vi "PC-Main.vi"() -> ()   [LabVIEW 2017]
doc: "The PC-Based PC-Main programme is a TCP/IP capable controller design to connect to the MR-Main programme in order to pass and receive data to simulate customisable cooling and emergency events via control of the MyRIO attached hardware, such as a PWM servo.\nIt has limited functionality if not connected to thge MR-Main programme."
uses:
  <vilib>/vision/Image Controls.llb/IMAQ Image.ctl
panel:
  out "Temperature (C)":dbl(knob) scale=18.0..30.0 scale format="%#.2g"
  out "Console":string
  out "Cool System Off Log":bool
  out "Z-Value\n(Debug)":dbl
  out "Y-Value\n(Debug":dbl
  out "X-Value\n(Debug)":dbl
  out "High Temp Log":bool
  out "Cool System On Log":bool
  out "Cool 4 Log":bool
  out "Cool 3 Log":bool
  out "Cool 2 Log":bool
  out "Cool 1 Log":bool
  out "Destroyed Log":bool
  out "Local Log":bool
  out "Moved Log":bool
  out "Disconnect Log":bool
  out "Connection Log":bool
  out "Nom Temp Log":bool
  out "Event Status\n(Debug)":u8
  out "User Level\n(Debug)":i32
  out "Local Request":bool
  out "Self Destruct":bool
  out "Master Warning":bool
  out "Cooling System":string
  in  "Auth":bool
  in  "Auth 2":bool
  in  "Authorise\nMovement (Debug)":bool
  out "Image":T1(plugin-control)
  out "Connected":bool
  out "Watchdog\n(Debug)":u8
  out "Net Error Source\n(Debug)":string
  out "Net Error Code\n(Debug)":i32
  out "Net Error Status\n(Debug)":bool
  in  "Quit":bool
  out "Handler Error Code\n(Debug)":i32
  in  "Cooling\nSwitch":bool
  out "Status System":timestamp format="%<%H:%M:%S\n%Y/%m/%d>T"
  out "Cooling Event Array\n(Debug)":bool[](array[boolean])
  out "Data Size\n(Debug)":i32
  out "String Length\n(Debug)":i32
  out "Cooling System Status":bool
  out "Cool Ind 4":bool
  out "Cool Ind 3":bool
  out "Cool Ind 2":bool
  out "Cool Ind 1":bool
  in  "Log Off":bool
  out "Movement":cluster{dbl, dbl, dbl}(graph)
  out "User Status":string
  in  "Password Match\n(Debug)":string[](array[string])
  in  "User Type\n(Debug)":string[](array[string])
  in  "Login":bool
  in  "Cooling 4 Off":timestamp format="%<%H:%M:%S>T"
  in  "Cooling 4 On":timestamp format="%<%H:%M:%S>T"
  in  "Cooling 3 Off":timestamp format="%<%H:%M:%S>T"
  in  "Cooling 3 On":timestamp format="%<%H:%M:%S>T"
  in  "Cooling 2 Off":timestamp format="%<%H:%M:%S>T"
  in  "Cooling 2 On":timestamp format="%<%H:%M:%S>T"
  in  "Cooling 1 Off":timestamp format="%<%H:%M:%S>T"
  in  "Cooling 1 On":timestamp format="%<%H:%M:%S>T"
  in  "Password":string
  in  "Username":string
  out "System Status":string
  out "Emergency Cooling":bool
  out "Safe System Temperature":bool
  # "Sensor System"
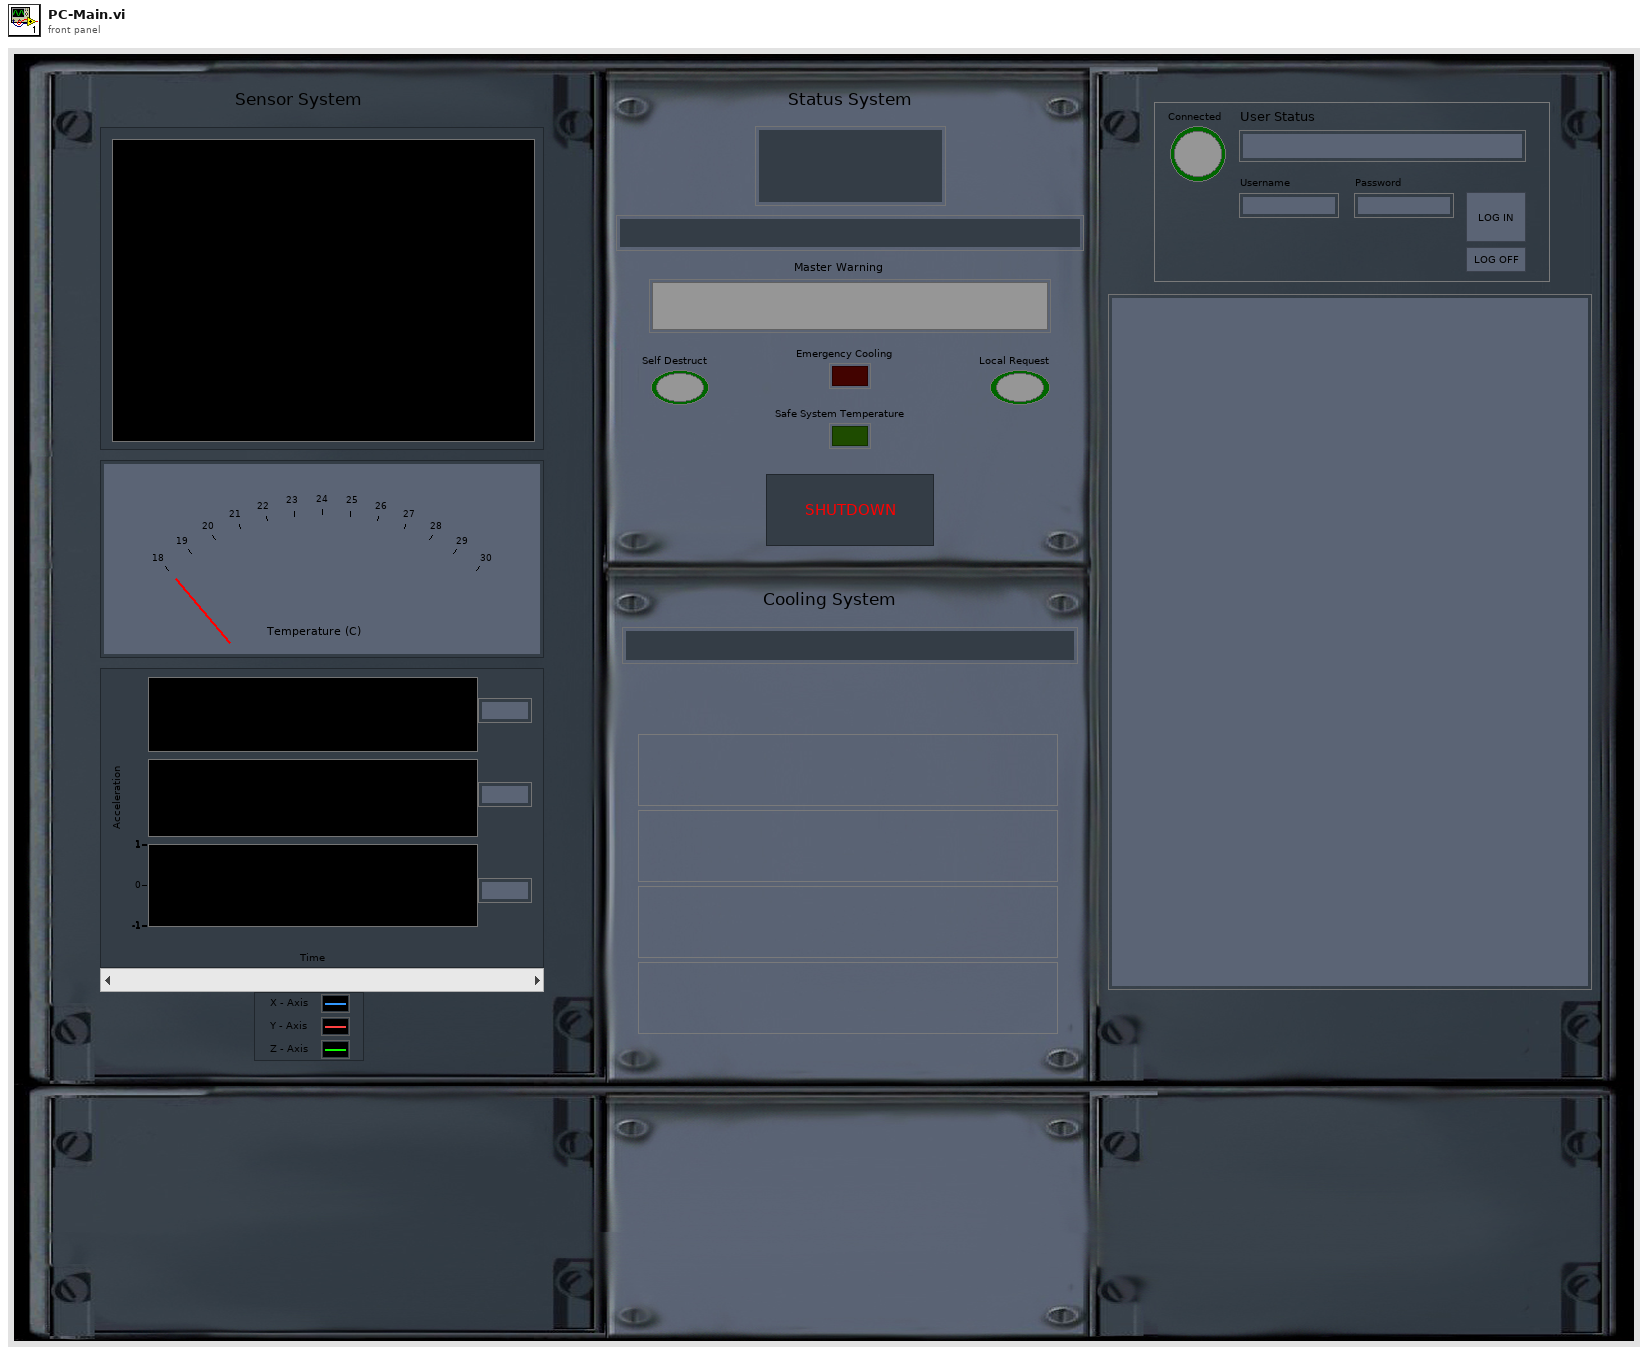
[diagram p1: front panel]
types:
  T1 = typedef "IMAQ Image.ctl" = refnum<image>
  T2 = cluster{"Numeric":dbl, "Knob":dbl, "Knob 2":dbl, "Knob 3":dbl, bool, "bytes to read":u8, "bytes to read 2":u8}
  T3 = cluster{"Numeric":dbl, "Numeric":dbl, "Numeric":dbl}
  T4 = cluster{"Cool Ind 1":bool, "Cool Ind 2":bool, "Cool Ind 3":bool, "Cool Ind 4":bool, bool, dbl, "Authorise\nMovement (Debug)":bool}
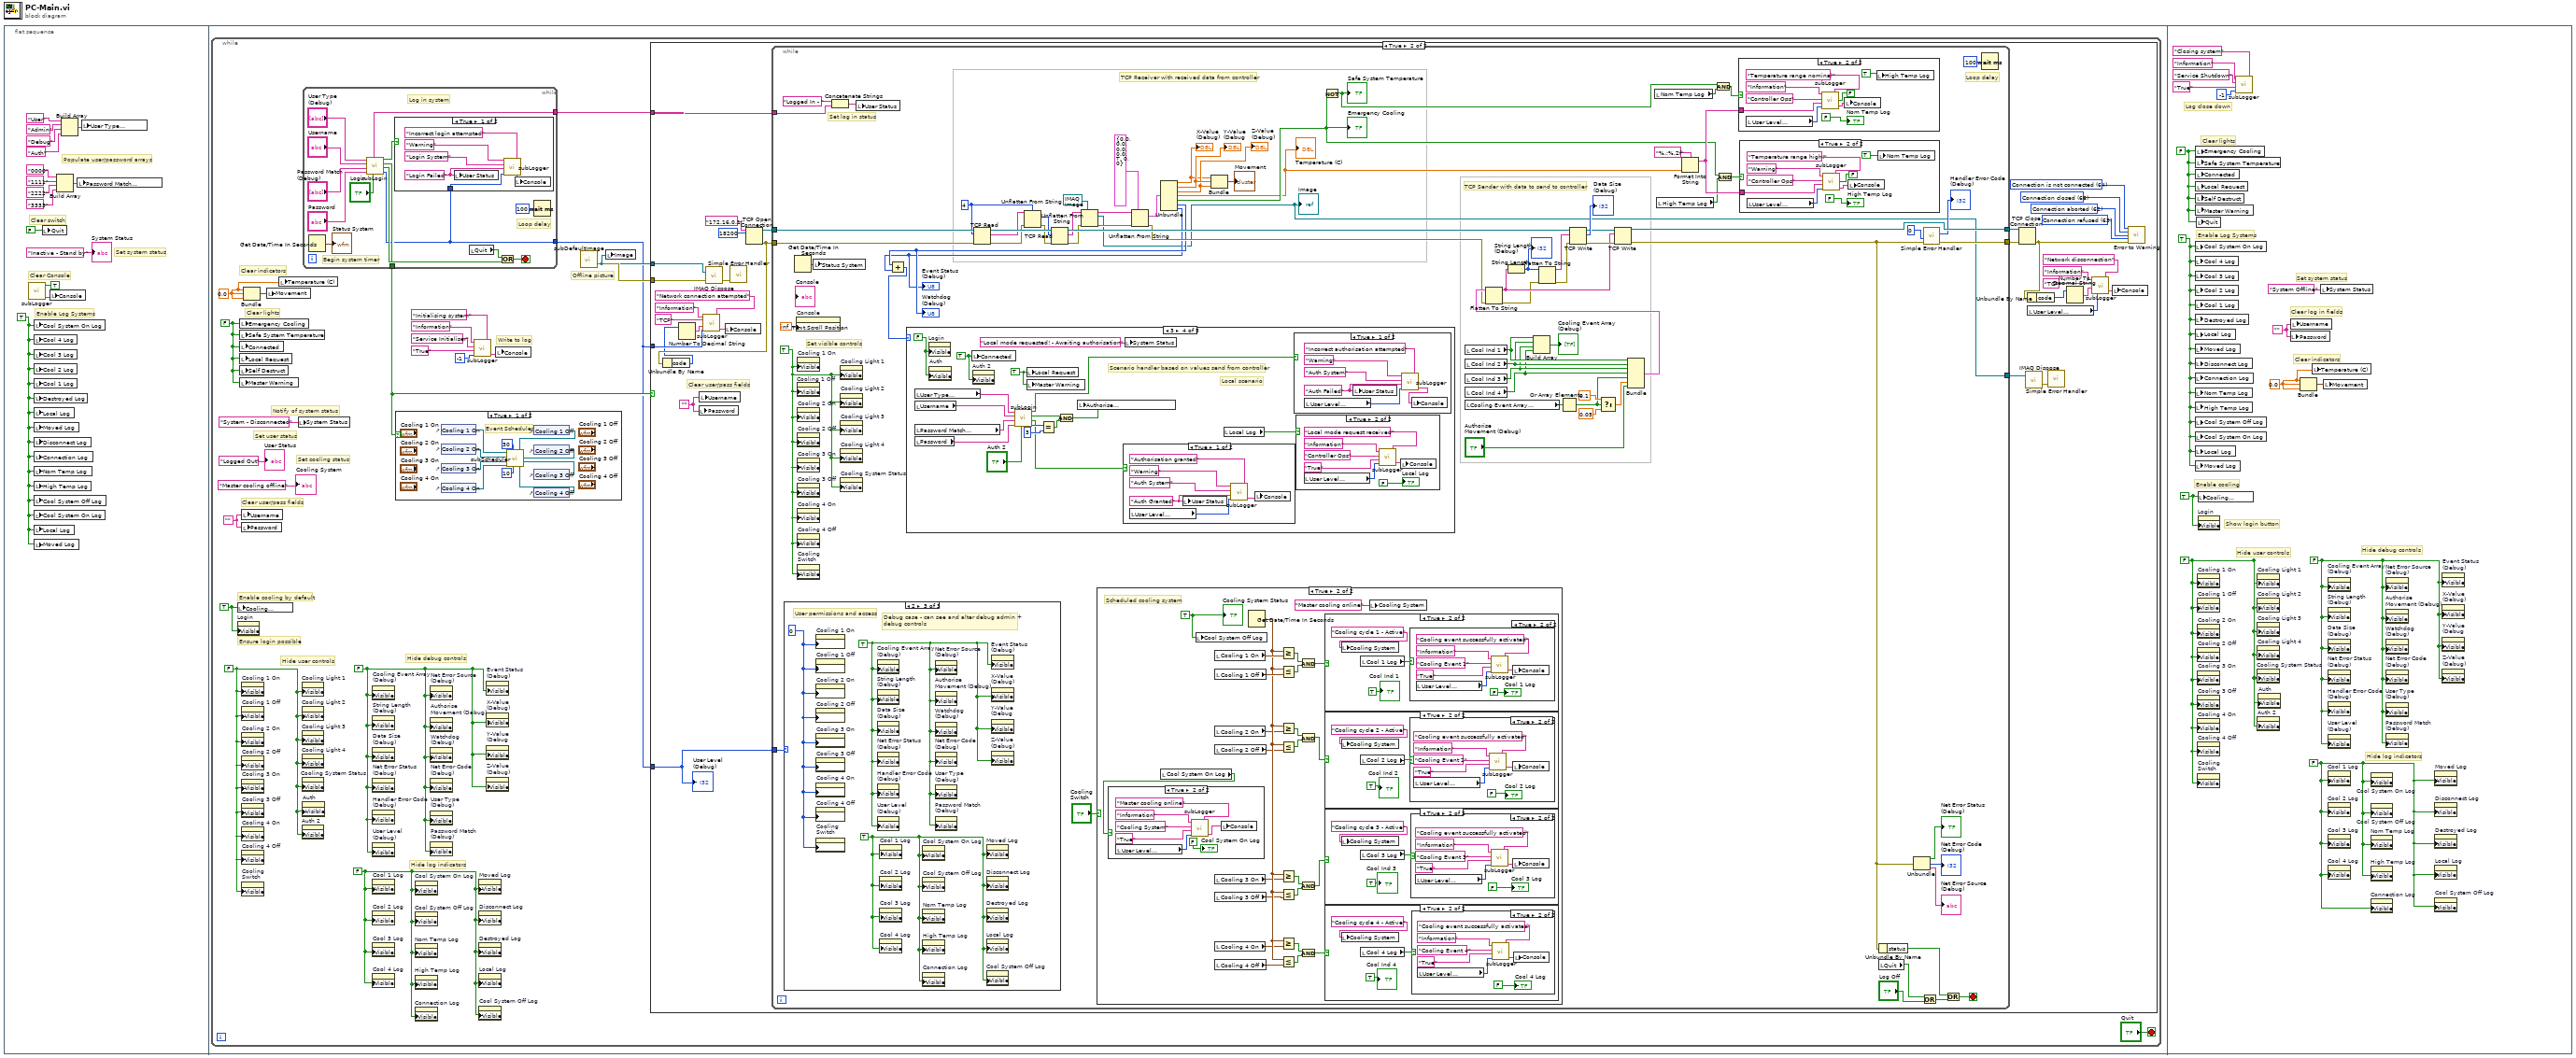
[diagram p0: block diagram]
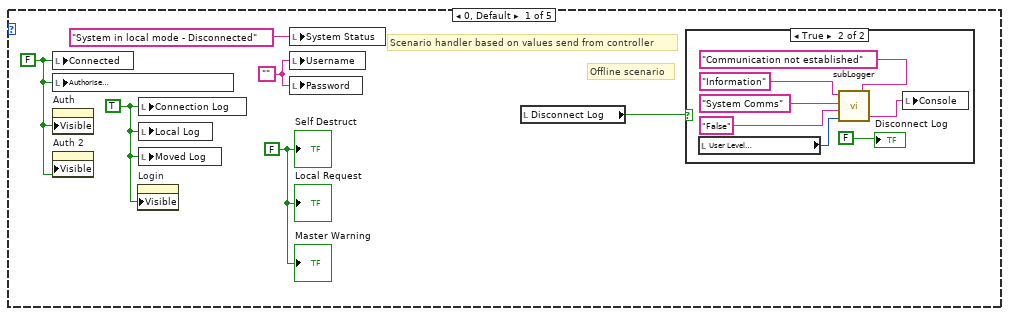
[diagram p7: hidden frame]
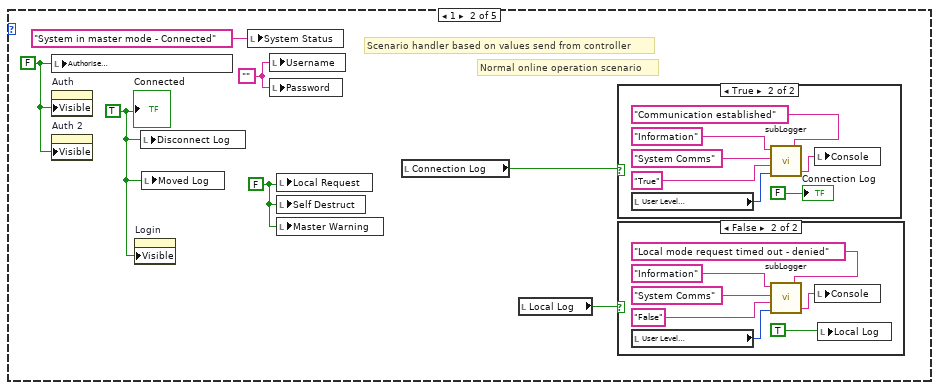
[diagram p9: hidden frame]
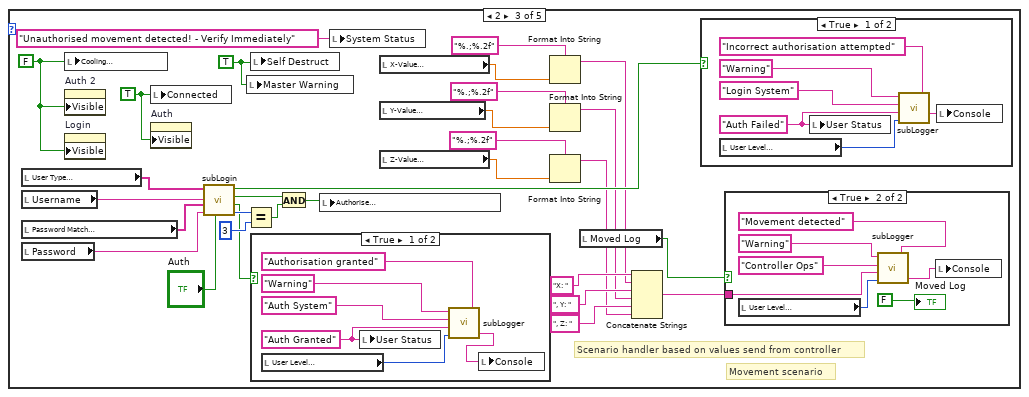
[diagram p12: hidden frame]
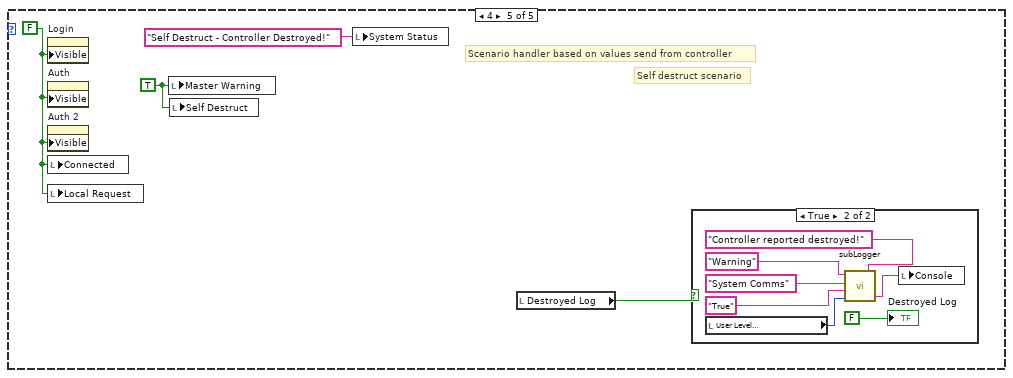
[diagram p19: hidden frame]
diagram:
  n1 = flat-sequence {
    frame #0 {
      w3 = TRUE
      # "Clear Console"
      # "Enable Log Systems"
      # "Set system status"
      # "Clear switch"
      # "Populate user/password arrays"
      n2 = call "subLogger.vi"("Clear Flag"=TRUE) -> ("To Screen"=w2:string)  [unwired: 5 in]
      n3 = local write "Cool System On Log"(w3) -> ()
      n4 = local write "Cool 4 Log"(w3) -> ()
      n5 = local write "Cool 3 Log"(w3) -> ()
      n6 = local write "Cool 2 Log"(w3) -> ()
      n7 = local write "Cool 1 Log"(w3) -> ()
      n8 = local write "Destroyed Log"(w3) -> ()
      n9 = local write "Local Log"(w3) -> ()
      n10 = local write "Moved Log"(w3) -> ()
      n11 = local write "Disconnect Log"(w3) -> ()
      n12 = local write "Connection Log"(w3) -> ()
      n13 = local write "Nom Temp Log"(w3) -> ()
      n14 = local write "High Temp Log"(w3) -> ()
      n15 = local write "Cool System Off Log"(w3) -> ()
      n16 = local write "Cool System On Log"(w3) -> ()
      n17 = local write "Local Log"(w3) -> ()
      n18 = local write "Moved Log"(w3) -> ()
      n19 = local write "Quit"(FALSE) -> ()
      n20 = local write "Console"(w2) -> ()
      n21 = Build Array("0000", "1111", "2222", "3333") -> (w15:string[])
      n22 = Build Array("User", "Admin", "Debug", "Auth") -> (w14:string[])
      n23 = local write "Password Match\n(Debug)"(w15) -> ()
      n24 = local write "User Type\n(Debug)"(w14) -> ()
      "System Status" <- "Inactive - Stand by"
    }
    frame #1 {
      n25 = while {
        stop <- "Quit" stop-if-true
        w17 = FALSE
        w18 = FALSE
        w33 = ""
        w16 = 0.0 ("Numeric")
        w27 = FALSE
        w31 = TRUE
        w19 = FALSE
        # "Offline picture"
        # "Hide log indicators"
        # "Hide debug controls"
        # "Write to log"
        # "Set cooling status"
        # "Ensure login possible"
        # "Notify of system status"
        # "Clear user/pass fields"
        # "Clear lights"
        # "Clear indicators"
        # "Enable cooling by default"
        # "Set user status"
        # "Hide user controls"
        n26 = local write "Cooling\nSwitch"(w31) -> ()
        n27 = property on="Login" class="Bool"("Visible"=w31) -> ()  [unwired: 2 in, 2 out]
        n28 = local write "Emergency Cooling"(w27) -> ()
        n29 = local write "Safe System Temperature"(w27) -> ()
        n30 = local write "Connected"(w27) -> ()
        n31 = local write "Local Request"(w27) -> ()
        n32 = local write "Self Destruct"(w27) -> ()
        n33 = local write "Master Warning"(w27) -> ()
        n34 = local write "Username"(w33) -> ()
        n35 = local write "Password"(w33) -> ()
        n36 = property on="Cooling 1 On" class="AbsTime (strict)"("Visible"=w19) -> ()  [unwired: 2 in, 2 out]
        n37 = property on="Cooling 1 Off" class="AbsTime (strict)"("Visible"=w19) -> ()  [unwired: 2 in, 2 out]
        n38 = property on="Cooling 2 On" class="AbsTime (strict)"("Visible"=w19) -> ()  [unwired: 2 in, 2 out]
        n39 = property on="Cooling 2 Off" class="AbsTime (strict)"("Visible"=w19) -> ()  [unwired: 2 in, 2 out]
        n40 = property on="Cooling 3 On" class="AbsTime (strict)"("Visible"=w19) -> ()  [unwired: 2 in, 2 out]
        n41 = property on="Cooling 3 Off" class="AbsTime (strict)"("Visible"=w19) -> ()  [unwired: 2 in, 2 out]
        n42 = property on="Cooling 4 On" class="AbsTime (strict)"("Visible"=w19) -> ()  [unwired: 2 in, 2 out]
        n43 = property on="Cooling 4 Off" class="AbsTime (strict)"("Visible"=w19) -> ()  [unwired: 2 in, 2 out]
        n44 = property on="Cooling\nSwitch" class="Bool (strict)"("Visible"=w19) -> ()  [unwired: 2 in, 2 out]
        n45 = Bundle("Numeric"=w16, "Numeric"=w16, "Numeric"=w16) -> (w34:T3)  [unwired: 1 in]
        n46 = local write "Movement"(w34) -> ()
        n47 = local write "Temperature (C)"(w16) -> ()
        n48 = local write "System Status"("System - Disconnected") -> ()
        n49 = property on="Cooling Light 1" class="Bool (strict)"("Visible"=w19) -> ()  [unwired: 2 in, 2 out]
        n50 = property on="Cooling Light 2" class="Bool (strict)"("Visible"=w19) -> ()  [unwired: 2 in, 2 out]
        n51 = property on="Cooling Light 3" class="Bool (strict)"("Visible"=w19) -> ()  [unwired: 2 in, 2 out]
        n52 = property on="Cooling Light 4" class="Bool (strict)"("Visible"=w19) -> ()  [unwired: 2 in, 2 out]
        n53 = property on="Cooling System Status" class="Bool (strict)"("Visible"=w19) -> ()  [unwired: 2 in, 2 out]
        n54 = property on="Auth 2" class="Bool"("Visible"=w19) -> ()  [unwired: 2 in, 2 out]
        n55 = property on="Auth" class="Bool"("Visible"=w19) -> ()  [unwired: 2 in, 2 out]
        n56 = while {
          tunnel: [w50] -> w26
          tunnel: [w56] -> w37
          tunnel: [w59] -> w38
          stop <- w62 stop-if-true
          # "Log in system"
          # "Loop delay"
          # "Begin system timer"
          n57 = Get Date/Time In Seconds() -> (seconds since 1Jan1904=→"Status System":timestamp)
          n58 = call "subLogin.vi"("Login Button"="Login", "Password Entry"="Password", "Password Array"="Password Match\n(Debug)", "User Entry"="Username", "User Array"="User Type\n(Debug)") -> ("Array Index No"=w50:i32, "If Correct 2"=w57:bool, "If Correct 1"=w56:bool, "If Incorrect"=w58:bool, "Username Out"=w59:string)
          n59 = case shown="True" w58 {
            tunnel: w50 -> [w65 _]
            frame True {
              w66 = "Login Failed"
              n60 = local write "User Status"(w66) -> ()
              n61 = call "subLogger.vi"("Description"="Incorrect login attempted", "User Level"=w65, "Value"=w66, "Location"="Login System", "Level"="Warning") -> ("To Screen"=w63:string)  [unwired: 1 in]
              n62 = local write "Console"(w63) -> ()
            }
            frame False {
            }
          }
          n63 = local read "Quit"() -> (w61:bool)
          n64 = Or(x=w61, y=w57) -> (x .or. y?=w62:bool)
          n65 = Wait (ms)(milliseconds to wait=u32 100) -> ()  [unwired: 1 out]
        }
        n66 = property on="Cooling Event Array\n(Debug)" class="Arr (strict)"("Visible"=w17) -> ()  [unwired: 2 in, 2 out]
        n67 = property on="String Length\n(Debug)" class="DigNum (strict)"("Visible"=w17) -> ()  [unwired: 2 in, 2 out]
        n68 = property on="Data Size\n(Debug)" class="DigNum (strict)"("Visible"=w17) -> ()  [unwired: 2 in, 2 out]
        n69 = property on="Net Error Status\n(Debug)" class="Bool (strict)"("Visible"=w17) -> ()  [unwired: 2 in, 2 out]
        n70 = property on="Handler Error Code\n(Debug)" class="DigNum (strict)"("Visible"=w17) -> ()  [unwired: 2 in, 2 out]
        n71 = property on="User Level\n(Debug)" class="DigNum (strict)"("Visible"=w17) -> ()  [unwired: 2 in, 2 out]
        n72 = property on="Cool 1 Log" class="Bool (strict)"("Visible"=w18) -> ()  [unwired: 2 in, 2 out]
        n73 = property on="Cool 2 Log" class="Bool (strict)"("Visible"=w18) -> ()  [unwired: 2 in, 2 out]
        n74 = property on="Cool 3 Log" class="Bool (strict)"("Visible"=w18) -> ()  [unwired: 2 in, 2 out]
        n75 = property on="Cool 4 Log" class="Bool (strict)"("Visible"=w18) -> ()  [unwired: 2 in, 2 out]
        n76 = case shown="True" w37 {
          frame True {
            # "Event Scheduler"
            n77 = control-ref of="Cooling 1 On"() -> (w42:refnum<vi>)
            n78 = control-ref of="Cooling 2 On"() -> (w41:refnum<vi>)
            n79 = control-ref of="Cooling 3 On"() -> (w40:refnum<vi>)
            n80 = control-ref of="Cooling 4 On"() -> (w39:refnum<vi>)
            n81 = control-ref of="Cooling 1 Off"() -> (w46:refnum<vi>)
            n82 = control-ref of="Cooling 2 Off"() -> (w45:refnum<vi>)
            n83 = control-ref of="Cooling 3 Off"() -> (w44:refnum<vi>)
            n84 = control-ref of="Cooling 4 Off"() -> (w43:refnum<vi>)
            n85 = call "subScheduler.vi"("Cooling 4 Off"=w43, "Cooling 3 Off"=w44, "Cooling 2 Off"=w45, "Cooling 1 Off"=w46, "Deactivate Offset"=10, "Activate Offset"=30, "Cooling 4 On"=w39, "Cooling 3 On"=w40, "Cooling 2 On"=w41, "Cooling 1 On"=w42) -> ()
          }
          frame False {
            # "Event Scheduler"
          }
        }
        n86 = property on="Cool System On Log" class="Bool (strict)"("Visible"=w18) -> ()  [unwired: 2 in, 2 out]
        n87 = property on="Cool System Off Log" class="Bool (strict)"("Visible"=w18) -> ()  [unwired: 2 in, 2 out]
        n88 = property on="Nom Temp Log" class="Bool (strict)"("Visible"=w18) -> ()  [unwired: 2 in, 2 out]
        n89 = property on="High Temp Log" class="Bool (strict)"("Visible"=w18) -> ()  [unwired: 2 in, 2 out]
        n90 = property on="Connection Log" class="Bool (strict)"("Visible"=w18) -> ()  [unwired: 2 in, 2 out]
        n91 = property on="Net Error Source\n(Debug)" class="Str"("Visible"=w17) -> ()  [unwired: 2 in, 2 out]
        n92 = property on="Authorise\nMovement (Debug)" class="Bool (strict)"("Visible"=w17) -> ()  [unwired: 2 in, 2 out]
        n93 = property on="Watchdog\n(Debug)" class="DigNum (strict)"("Visible"=w17) -> ()  [unwired: 2 in, 2 out]
        n94 = property on="Net Error Code\n(Debug)" class="DigNum (strict)"("Visible"=w17) -> ()  [unwired: 2 in, 2 out]
        n95 = property on="User Type\n(Debug)" class="Arr (strict)"("Visible"=w17) -> ()  [unwired: 2 in, 2 out]
        n96 = property on="Password Match\n(Debug)" class="Arr (strict)"("Visible"=w17) -> ()  [unwired: 2 in, 2 out]
        n97 = call "subLogger.vi"("Description"="Initialising system", "User Level"=-1, "Value"="True", "Location"="Service Initialiser", "Level"="Information") -> ("To Screen"=w25:string)  [unwired: 1 in]
        n98 = property on="Moved Log" class="Bool (strict)"("Visible"=w18) -> ()  [unwired: 2 in, 2 out]
        n99 = property on="Disconnect Log" class="Bool (strict)"("Visible"=w18) -> ()  [unwired: 2 in, 2 out]
        n100 = property on="Destroyed Log" class="Bool (strict)"("Visible"=w18) -> ()  [unwired: 2 in, 2 out]
        n101 = property on="Local Log" class="Bool (strict)"("Visible"=w18) -> ()  [unwired: 2 in, 2 out]
        n102 = property on="Cool System Off Log" class="Bool (strict)"("Visible"=w18) -> ()  [unwired: 2 in, 2 out]
        n103 = property on="Event Status\n(Debug)" class="DigNum (strict)"("Visible"=w17) -> ()  [unwired: 2 in, 2 out]
        n104 = property on="X-Value\n(Debug)" class="DigNum (strict)"("Visible"=w17) -> ()  [unwired: 2 in, 2 out]
        n105 = property on="Y-Value\n(Debug" class="DigNum (strict)"("Visible"=w17) -> ()  [unwired: 2 in, 2 out]
        n106 = property on="Z-Value\n(Debug)" class="DigNum (strict)"("Visible"=w17) -> ()  [unwired: 2 in, 2 out]
        n107 = local write "Console"(w25) -> ()
        n108 = call "subDefaultImage.vi"() -> ("error out"=w29:errorcluster, "Image"=w28:T1)  [unwired: 2 in]
        n109 = local write "Image"(w28) -> ()
        n110 = case shown="True" w37 {
          tunnel: w26 -> [_ w81]
          tunnel: w38 -> [_ w93]
          tunnel: w29 -> [_ w89]
          tunnel: w28 -> [_ w87]
          tunnel: w26 -> [_ w80]
          frame False {
          }
          frame True {
            w91 = ""
            w92 = 63 items=["No Error", "Argument Error", "Memory Full", "Out of Zone", "End of File", "File Already Open", "Generic File IO Error", "File Not Found", "File Permission Error", "Disk Full", "Duplicate Path", "Too Many Files Open", "Not Enabled", "Resource File Not Found", "Cannot Add Resource", "Resource Not Found", "Image Not Found", "Image Memory Error", "Pen Does Not Exist", "Config Bad Type", "Config Token Not Found", "Config Parse Error", "Config Memory Error", "Bad External Code Format", "Bad External Code Offset", "External Code Not Present", "Null Window", "Destroy Window Mixup", "Null Menu", "Print Aborted", "Bad Print Record", "Print Driver Error", "Windows Error During Print", "Memory Error During Print", "Print Dialog Error", "Generic Print Error", "Invalid Device Refnum", "Device Not Found", "Device Parameter Error", "Device Unit Error", "Can't Open Device", "Device Call Aborted", "Generic Error", "Cancelled By User", "Object ID Too Low", "Object ID Too High", "Object Not In Heap", "Unknown Heap", "Bad DefProc ID", "DefProc Not In Table", "Message Out Of Range", "Null Method", "Unknown Message", "Manager Call Not Supported", "Bad address", "Connection In progress", "Connection timed out", "Connection is already in progress", "Network attribute not supported", "Network error", "Address in use", "System out of memory", "Connection aborted", "Connection refused", "Connection is not connected", "Connection is already connected", "Connection closed", "Initialize error (interapplication manager)", "Bad occurrence", "Wait on unbound occurrence handler", "Occurrence queue overflow", "Bad path", "Semaphore not signaled", "Unrecognized type (interapplication manager)"] ("4th Error to Convert")
            w96 = 62 items=["No Error", "Argument Error", "Memory Full", "Out of Zone", "End of File", "File Already Open", "Generic File IO Error", "File Not Found", "File Permission Error", "Disk Full", "Duplicate Path", "Too Many Files Open", "Not Enabled", "Resource File Not Found", "Cannot Add Resource", "Resource Not Found", "Image Not Found", "Image Memory Error", "Pen Does Not Exist", "Config Bad Type", "Config Token Not Found", "Config Parse Error", "Config Memory Error", "Bad External Code Format", "Bad External Code Offset", "External Code Not Present", "Null Window", "Destroy Window Mixup", "Null Menu", "Print Aborted", "Bad Print Record", "Print Driver Error", "Windows Error During Print", "Memory Error During Print", "Print Dialog Error", "Generic Print Error", "Invalid Device Refnum", "Device Not Found", "Device Parameter Error", "Device Unit Error", "Can't Open Device", "Device Call Aborted", "Generic Error", "Cancelled By User", "Object ID Too Low", "Object ID Too High", "Object Not In Heap", "Unknown Heap", "Bad DefProc ID", "DefProc Not In Table", "Message Out Of Range", "Null Method", "Unknown Message", "Manager Call Not Supported", "Bad address", "Connection In progress", "Connection timed out", "Connection is already in progress", "Network attribute not supported", "Network error", "Address in use", "System out of memory", "Connection aborted", "Connection refused", "Connection is not connected", "Connection is already connected", "Connection closed", "Initialize error (interapplication manager)", "Bad occurrence", "Wait on unbound occurrence handler", "Occurrence queue overflow", "Bad path", "Semaphore not signaled", "Unrecognized type (interapplication manager)"] ("3rd Error to Convert")
            w97 = 66 items=["No Error", "Argument Error", "Memory Full", "Out of Zone", "End of File", "File Already Open", "Generic File IO Error", "File Not Found", "File Permission Error", "Disk Full", "Duplicate Path", "Too Many Files Open", "Not Enabled", "Resource File Not Found", "Cannot Add Resource", "Resource Not Found", "Image Not Found", "Image Memory Error", "Pen Does Not Exist", "Config Bad Type", "Config Token Not Found", "Config Parse Error", "Config Memory Error", "Bad External Code Format", "Bad External Code Offset", "External Code Not Present", "Null Window", "Destroy Window Mixup", "Null Menu", "Print Aborted", "Bad Print Record", "Print Driver Error", "Windows Error During Print", "Memory Error During Print", "Print Dialog Error", "Generic Print Error", "Invalid Device Refnum", "Device Not Found", "Device Parameter Error", "Device Unit Error", "Can't Open Device", "Device Call Aborted", "Generic Error", "Cancelled By User", "Object ID Too Low", "Object ID Too High", "Object Not In Heap", "Unknown Heap", "Bad DefProc ID", "DefProc Not In Table", "Message Out Of Range", "Null Method", "Unknown Message", "Manager Call Not Supported", "Bad address", "Connection In progress", "Connection timed out", "Connection is already in progress", "Network attribute not supported", "Network error", "Address in use", "System out of memory", "Connection aborted", "Connection refused", "Connection is not connected", "Connection is already connected", "Connection closed", "Initialize error (interapplication manager)", "Bad occurrence", "Wait on unbound occurrence handler", "Occurrence queue overflow", "Bad path", "Semaphore not signaled", "Unrecognized type (interapplication manager)"] ("2nd Error to Convert")
            w98 = 64 items=["No Error", "Argument Error", "Memory Full", "Out of Zone", "End of File", "File Already Open", "Generic File IO Error", "File Not Found", "File Permission Error", "Disk Full", "Duplicate Path", "Too Many Files Open", "Not Enabled", "Resource File Not Found", "Cannot Add Resource", "Resource Not Found", "Image Not Found", "Image Memory Error", "Pen Does Not Exist", "Config Bad Type", "Config Token Not Found", "Config Parse Error", "Config Memory Error", "Bad External Code Format", "Bad External Code Offset", "External Code Not Present", "Null Window", "Destroy Window Mixup", "Null Menu", "Print Aborted", "Bad Print Record", "Print Driver Error", "Windows Error During Print", "Memory Error During Print", "Print Dialog Error", "Generic Print Error", "Invalid Device Refnum", "Device Not Found", "Device Parameter Error", "Device Unit Error", "Can't Open Device", "Device Call Aborted", "Generic Error", "Cancelled By User", "Object ID Too Low", "Object ID Too High", "Object Not In Heap", "Unknown Heap", "Bad DefProc ID", "DefProc Not In Table", "Message Out Of Range", "Null Method", "Unknown Message", "Manager Call Not Supported", "Bad address", "Connection In progress", "Connection timed out", "Connection is already in progress", "Network attribute not supported", "Network error", "Address in use", "System out of memory", "Connection aborted", "Connection refused", "Connection is not connected", "Connection is already connected", "Connection closed", "Initialize error (interapplication manager)", "Bad occurrence", "Wait on unbound occurrence handler", "Occurrence queue overflow", "Bad path", "Semaphore not signaled", "Unrecognized type (interapplication manager)"] ("1st Error to Convert")
            # "Clear user/pass fields"
            n111 = local write "Password"(w91) -> ()
            n112 = local write "Username"(w91) -> ()
            n113 = call "IMAQ Dispose"("Image"=w87, "error in (no error)"=w89) -> ("error out"=w88:errorcluster)  [unwired: 4 in]
            n114 = call <vilib>:"Simple Error Handler.vi"("error in (no error)"=w88) -> ()  [unwired: 1 in, 8 out]
            n115 = TCP Open Connection(address="172.16.0.1", remote port or service name=u16 18200) -> (connection ID=w99:refnum<k5>, error out=w70:errorcluster)  [unwired: 1 in, 2 out]
            n116 = Unbundle By Name(w70) -> ("code"=w69:i32)
            n117 = Number To Decimal String(number=w69) -> (decimal integer string=w85:string)  [unwired: 1 in]
            n118 = call "subLogger.vi"("Description"="Network connection attempted", "User Level"=w80, "Value"=w85, "Location"="TCP", "Level"="Information") -> ("To Screen"=w72:string)  [unwired: 1 in]
            n119 = local write "Console"(w72) -> ()
            n120 = while {
              tunnel: w99 -> [w148]
              tunnel: w70 -> [w147]
              tunnel: [w152] -> w95
              tunnel: [w151] -> w94
              tunnel: w81 -> [w165]
              tunnel: w93 -> [w155]
              tunnel: [w103] -> w90
              stop <- w138 stop-if-true
              w137 = 4 ("bytes to read")
              w153 = TRUE
              # "TCP Sender with data to send to controller"
              # "TCP Receiver with received data from controller"
              # "Loop delay"
              # "Set log in status"
              # "Set visible controls"
              n121 = case shown="2" w165 {
                frame 0 {
                  w412 = u8 2
                  # "User permissions and access"
                  # "Standard user case - preset cooling, no\nability to change, monitor only"
                  n122 = property on="Cooling 1 On" class="AbsTime (strict)"("DisabledEnum"=w412) -> ()  [unwired: 2 in, 2 out]
                  n123 = property on="Cooling 1 Off" class="AbsTime (strict)"("DisabledEnum"=w412) -> ()  [unwired: 2 in, 2 out]
                  n124 = property on="Cooling 2 On" class="AbsTime (strict)"("DisabledEnum"=w412) -> ()  [unwired: 2 in, 2 out]
                  n125 = property on="Cooling 2 Off" class="AbsTime (strict)"("DisabledEnum"=w412) -> ()  [unwired: 2 in, 2 out]
                  n126 = property on="Cooling 3 On" class="AbsTime (strict)"("DisabledEnum"=w412) -> ()  [unwired: 2 in, 2 out]
                  n127 = property on="Cooling 3 Off" class="AbsTime (strict)"("DisabledEnum"=w412) -> ()  [unwired: 2 in, 2 out]
                  n128 = property on="Cooling 4 On" class="AbsTime (strict)"("DisabledEnum"=w412) -> ()  [unwired: 2 in, 2 out]
                  n129 = property on="Cooling 4 Off" class="AbsTime (strict)"("DisabledEnum"=w412) -> ()  [unwired: 2 in, 2 out]
                  n130 = property on="Cooling\nSwitch" class="Bool (strict)"("DisabledEnum"=w412) -> ()  [unwired: 2 in, 2 out]
                }
                frame 1, Default {
                  w413 = 0
                  # "User permissions and access"
                  # "Administrator case - Can change schedule"
                  n131 = property on="Cooling 1 On" class="AbsTime (strict)"("DisabledEnum"=w413) -> ()  [unwired: 2 in, 2 out]
                  n132 = property on="Cooling 1 Off" class="AbsTime (strict)"("DisabledEnum"=w413) -> ()  [unwired: 2 in, 2 out]
                  n133 = property on="Cooling 2 On" class="AbsTime (strict)"("DisabledEnum"=w413) -> ()  [unwired: 2 in, 2 out]
                  n134 = property on="Cooling 2 Off" class="AbsTime (strict)"("DisabledEnum"=w413) -> ()  [unwired: 2 in, 2 out]
                  n135 = property on="Cooling 3 On" class="AbsTime (strict)"("DisabledEnum"=w413) -> ()  [unwired: 2 in, 2 out]
                  n136 = property on="Cooling 3 Off" class="AbsTime (strict)"("DisabledEnum"=w413) -> ()  [unwired: 2 in, 2 out]
                  n137 = property on="Cooling 4 On" class="AbsTime (strict)"("DisabledEnum"=w413) -> ()  [unwired: 2 in, 2 out]
                  n138 = property on="Cooling 4 Off" class="AbsTime (strict)"("DisabledEnum"=w413) -> ()  [unwired: 2 in, 2 out]
                  n139 = property on="Cooling\nSwitch" class="Bool (strict)"("DisabledEnum"=w413) -> ()  [unwired: 2 in, 2 out]
                }
                frame 2 {
                  w414 = TRUE
                  w415 = TRUE
                  w416 = 0
                  # "User permissions and access"
                  # "Debug case - can see and alter debug admin +\ndebug controls"
                  n140 = property on="Cooling 1 On" class="AbsTime (strict)"("DisabledEnum"=w416) -> ()  [unwired: 2 in, 2 out]
                  n141 = property on="Cooling 1 Off" class="AbsTime (strict)"("DisabledEnum"=w416) -> ()  [unwired: 2 in, 2 out]
                  n142 = property on="Cooling 2 On" class="AbsTime (strict)"("DisabledEnum"=w416) -> ()  [unwired: 2 in, 2 out]
                  n143 = property on="Cooling 2 Off" class="AbsTime (strict)"("DisabledEnum"=w416) -> ()  [unwired: 2 in, 2 out]
                  n144 = property on="Cooling 3 On" class="AbsTime (strict)"("DisabledEnum"=w416) -> ()  [unwired: 2 in, 2 out]
                  n145 = property on="Cooling 3 Off" class="AbsTime (strict)"("DisabledEnum"=w416) -> ()  [unwired: 2 in, 2 out]
                  n146 = property on="Cooling 4 On" class="AbsTime (strict)"("DisabledEnum"=w416) -> ()  [unwired: 2 in, 2 out]
                  n147 = property on="Cooling 4 Off" class="AbsTime (strict)"("DisabledEnum"=w416) -> ()  [unwired: 2 in, 2 out]
                  n148 = property on="Cooling\nSwitch" class="Bool (strict)"("DisabledEnum"=w416) -> ()  [unwired: 2 in, 2 out]
                  n149 = property on="Cooling Event Array\n(Debug)" class="Arr (strict)"("Visible"=w415) -> ()  [unwired: 2 in, 2 out]
                  n150 = property on="String Length\n(Debug)" class="DigNum (strict)"("Visible"=w415) -> ()  [unwired: 2 in, 2 out]
                  n151 = property on="Data Size\n(Debug)" class="DigNum (strict)"("Visible"=w415) -> ()  [unwired: 2 in, 2 out]
                  n152 = property on="Net Error Status\n(Debug)" class="Bool (strict)"("Visible"=w415) -> ()  [unwired: 2 in, 2 out]
                  n153 = property on="Handler Error Code\n(Debug)" class="DigNum (strict)"("Visible"=w415) -> ()  [unwired: 2 in, 2 out]
                  n154 = property on="User Level\n(Debug)" class="DigNum (strict)"("Visible"=w415) -> ()  [unwired: 2 in, 2 out]
                  n155 = property on="Cool 1 Log" class="Bool (strict)"("Visible"=w414) -> ()  [unwired: 2 in, 2 out]
                  n156 = property on="Cool 2 Log" class="Bool (strict)"("Visible"=w414) -> ()  [unwired: 2 in, 2 out]
                  n157 = property on="Cool 3 Log" class="Bool (strict)"("Visible"=w414) -> ()  [unwired: 2 in, 2 out]
                  n158 = property on="Cool 4 Log" class="Bool (strict)"("Visible"=w414) -> ()  [unwired: 2 in, 2 out]
                  n159 = property on="Cool System On Log" class="Bool (strict)"("Visible"=w414) -> ()  [unwired: 2 in, 2 out]
                  n160 = property on="Cool System Off Log" class="Bool (strict)"("Visible"=w414) -> ()  [unwired: 2 in, 2 out]
                  n161 = property on="Nom Temp Log" class="Bool (strict)"("Visible"=w414) -> ()  [unwired: 2 in, 2 out]
                  n162 = property on="High Temp Log" class="Bool (strict)"("Visible"=w414) -> ()  [unwired: 2 in, 2 out]
                  n163 = property on="Connection Log" class="Bool (strict)"("Visible"=w414) -> ()  [unwired: 2 in, 2 out]
                  n164 = property on="Net Error Source\n(Debug)" class="Str"("Visible"=w415) -> ()  [unwired: 2 in, 2 out]
                  n165 = property on="Authorise\nMovement (Debug)" class="Bool (strict)"("Visible"=w415) -> ()  [unwired: 2 in, 2 out]
                  n166 = property on="Watchdog\n(Debug)" class="DigNum (strict)"("Visible"=w415) -> ()  [unwired: 2 in, 2 out]
                  n167 = property on="Net Error Code\n(Debug)" class="DigNum (strict)"("Visible"=w415) -> ()  [unwired: 2 in, 2 out]
                  n168 = property on="User Type\n(Debug)" class="Arr (strict)"("Visible"=w415) -> ()  [unwired: 2 in, 2 out]
                  n169 = property on="Password Match\n(Debug)" class="Arr (strict)"("Visible"=w415) -> ()  [unwired: 2 in, 2 out]
                  n170 = property on="Moved Log" class="Bool (strict)"("Visible"=w414) -> ()  [unwired: 2 in, 2 out]
                  n171 = property on="Disconnect Log" class="Bool (strict)"("Visible"=w414) -> ()  [unwired: 2 in, 2 out]
                  n172 = property on="Destroyed Log" class="Bool (strict)"("Visible"=w414) -> ()  [unwired: 2 in, 2 out]
                  n173 = property on="Local Log" class="Bool (strict)"("Visible"=w414) -> ()  [unwired: 2 in, 2 out]
                  n174 = property on="Cool System Off Log" class="Bool (strict)"("Visible"=w414) -> ()  [unwired: 2 in, 2 out]
                  n175 = property on="Event Status\n(Debug)" class="DigNum (strict)"("Visible"=w415) -> ()  [unwired: 2 in, 2 out]
                  n176 = property on="X-Value\n(Debug)" class="DigNum (strict)"("Visible"=w415) -> ()  [unwired: 2 in, 2 out]
                  n177 = property on="Y-Value\n(Debug" class="DigNum (strict)"("Visible"=w415) -> ()  [unwired: 2 in, 2 out]
                  n178 = property on="Z-Value\n(Debug)" class="DigNum (strict)"("Visible"=w415) -> ()  [unwired: 2 in, 2 out]
                }
              }
              n179 = Get Date/Time In Seconds() -> (seconds since 1Jan1904=w117:timestamp)
              n180 = property on="Console" class="Str"("Text.Scroll Position"=inf) -> ()  [unwired: 2 in, 2 out]
              n181 = property on="Cooling 1 On" class="AbsTime (strict)"("Visible"=w153) -> ()  [unwired: 2 in, 2 out]
              n182 = property on="Cooling 1 Off" class="AbsTime (strict)"("Visible"=w153) -> ()  [unwired: 2 in, 2 out]
              n183 = property on="Cooling 2 On" class="AbsTime (strict)"("Visible"=w153) -> ()  [unwired: 2 in, 2 out]
              n184 = property on="Cooling 2 Off" class="AbsTime (strict)"("Visible"=w153) -> ()  [unwired: 2 in, 2 out]
              n185 = property on="Cooling 3 On" class="AbsTime (strict)"("Visible"=w153) -> ()  [unwired: 2 in, 2 out]
              n186 = property on="Cooling 3 Off" class="AbsTime (strict)"("Visible"=w153) -> ()  [unwired: 2 in, 2 out]
              n187 = property on="Cooling 4 On" class="AbsTime (strict)"("Visible"=w153) -> ()  [unwired: 2 in, 2 out]
              n188 = property on="Cooling 4 Off" class="AbsTime (strict)"("Visible"=w153) -> ()  [unwired: 2 in, 2 out]
              n189 = property on="Cooling\nSwitch" class="Bool (strict)"("Visible"=w153) -> ()  [unwired: 2 in, 2 out]
              n190 = local write "Status System"(w117) -> ()
              n191 = Concatenate Strings("Logged In - ", w155) -> (w157:string)
              n192 = property on="Cooling Light 1" class="Bool (strict)"("Visible"=w153) -> ()  [unwired: 2 in, 2 out]
              n193 = property on="Cooling Light 2" class="Bool (strict)"("Visible"=w153) -> ()  [unwired: 2 in, 2 out]
              n194 = property on="Cooling Light 3" class="Bool (strict)"("Visible"=w153) -> ()  [unwired: 2 in, 2 out]
              n195 = property on="Cooling Light 4" class="Bool (strict)"("Visible"=w153) -> ()  [unwired: 2 in, 2 out]
              n196 = property on="Cooling System Status" class="Bool (strict)"("Visible"=w153) -> ()  [unwired: 2 in, 2 out]
              n197 = local write "User Status"(w157) -> ()
              n198 = TCP Read(connection ID=w148, bytes to read=w137, error in (no error)=w147) -> (connection ID out=w176:refnum<k5>, data out=w136:string, error out=w135:errorcluster)  [unwired: 2 out]
              n199 = Unflatten From String(type=w137, binary string=w136, error in (no error)=w135) -> (value=w133:i32, error out=w134:errorcluster)  [unwired: 2 in, 1 out]
              n200 = TCP Read(connection ID=w176, bytes to read=w133, error in (no error)=w134) -> (connection ID out=w171:refnum<k5>, data out=w130:string, error out=w127:errorcluster)  [unwired: 2 out]
              n201 = Unflatten From String(type=T1 refnum ("Image"), binary string=w130, error in (no error)=w127) -> (rest of the binary string=w128:string, value=w103:T1, error out=w126:errorcluster)  [unwired: 2 in]
              "Image" <- w103
              n202 = case shown="True" "Cooling\nSwitch" {
                frame False {
                  w326 = TRUE
                  w328 = FALSE
                  # "Scheduled cooling system"
                  n203 = local write "Cool System On Log"(w326) -> ()
                  n204 = local write "Cool 1 Log"(w326) -> ()
                  n205 = local write "Cool 2 Log"(w326) -> ()
                  n206 = local write "Cool 3 Log"(w326) -> ()
                  n207 = local write "Cool 4 Log"(w326) -> ()
                  n208 = local read "Cool System Off Log"() -> (w327:bool)
                  n209 = case shown="True" w327 {
                    frame False {
                    }
                    frame True {
                      n210 = local read "User Level\n(Debug)"() -> (w333:i32)
                      n211 = call "subLogger.vi"("Description"="Master cooling offline", "User Level"=w333, "Value"="False", "Location"="Cooling System", "Level"="Warning") -> ("To Screen"=w330:string)  [unwired: 1 in]
                      n212 = local write "Console"(w330) -> ()
                      "Cool System Off Log" <- FALSE
                    }
                  }
                  n213 = local write "Cooling System"("Master cooling offline") -> ()
                  n214 = local write "Cooling System Status"(w328) -> ()
                  n215 = local write "Cool Ind 1"(w328) -> ()
                  n216 = local write "Cool Ind 2"(w328) -> ()
                  n217 = local write "Cool Ind 3"(w328) -> ()
                  n218 = local write "Cool Ind 4"(w328) -> ()
                }
                frame True {
                  w338 = TRUE
                  # "Scheduled cooling system"
                  n219 = local read "Cool System On Log"() -> (w337:bool)
                  n220 = case shown="True" w337 {
                    frame False {
                    }
                    frame True {
                      n221 = local read "User Level\n(Debug)"() -> (w363:i32)
                      n222 = call "subLogger.vi"("Description"="Master cooling online", "User Level"=w363, "Value"="True", "Location"="Cooling System", "Level"="Information") -> ("To Screen"=w361:string)  [unwired: 1 in]
                      n223 = local write "Console"(w361) -> ()
                      "Cool System On Log" <- FALSE
                    }
                  }
                  n224 = local write "Cool System Off Log"(w338) -> ()
                  n225 = local read "Cooling 1 On"() -> (w357:timestamp)
                  n226 = local read "Cooling 1 Off"() -> (w358:timestamp)
                  n227 = local read "Cooling 2 On"() -> (w349:timestamp)
                  n228 = local read "Cooling 2 Off"() -> (w348:timestamp)
                  n229 = local read "Cooling 3 On"() -> (w347:timestamp)
                  n230 = local read "Cooling 3 Off"() -> (w346:timestamp)
                  n231 = local read "Cooling 4 On"() -> (w345:timestamp)
                  n232 = local read "Cooling 4 Off"() -> (w344:timestamp)
                  n233 = Get Date/Time In Seconds() -> (seconds since 1Jan1904=w350:timestamp)
                  n234 = Greater Or Equal?(x=w350, y=w357) -> (x >= y?=w359:bool)
                  n235 = Less Or Equal?(x=w350, y=w358) -> (x <= y?=w360:bool)
                  n236 = Greater Or Equal?(x=w350, y=w349) -> (x >= y?=w356:bool)
                  n237 = Less Or Equal?(x=w350, y=w348) -> (x <= y?=w355:bool)
                  n238 = Greater Or Equal?(x=w350, y=w347) -> (x >= y?=w353:bool)
                  n239 = Less Or Equal?(x=w350, y=w346) -> (x <= y?=w354:bool)
                  n240 = Greater Or Equal?(x=w350, y=w345) -> (x >= y?=w352:bool)
                  n241 = Less Or Equal?(x=w350, y=w344) -> (x <= y?=w351:bool)
                  n242 = And(x=w359, y=w360) -> (x .and. y?=w343:bool)
                  n243 = And(x=w356, y=w355) -> (x .and. y?=w342:bool)
                  n244 = And(x=w353, y=w354) -> (x .and. y?=w341:bool)
                  n245 = And(x=w352, y=w351) -> (x .and. y?=w340:bool)
                  n246 = case shown="True" w343 {
                    frame False {
                      n247 = local write "Cool Ind 1"(FALSE) -> ()
                    }
                    frame True {
                      n248 = local write "Cooling System"("Cooling cycle 1 - Active") -> ()
                      n249 = local read "Cool 1 Log"() -> (w402:bool)
                      n250 = case shown="True" w402 {
                        frame False {
                        }
                        frame True {
                          n251 = local read "User Level\n(Debug)"() -> (w411:i32)
                          n252 = call "subLogger.vi"("Description"="Cooling event successfully activated", "User Level"=w411, "Value"="True", "Location"="Cooling Event 1", "Level"="Information") -> ("To Screen"=w405:string)  [unwired: 1 in]
                          n253 = local write "Console"(w405) -> ()
                          "Cool 1 Log" <- FALSE
                        }
                      }
                      "Cool Ind 1" <- TRUE
                    }
                  }
                  n254 = case shown="True" w342 {
                    frame False {
                      n255 = local write "Cool Ind 2"(FALSE) -> ()
                    }
                    frame True {
                      n256 = local write "Cooling System"("Cooling cycle 2 - Active") -> ()
                      n257 = local read "Cool 2 Log"() -> (w391:bool)
                      n258 = case shown="True" w391 {
                        frame False {
                        }
                        frame True {
                          n259 = local read "User Level\n(Debug)"() -> (w400:i32)
                          n260 = call "subLogger.vi"("Description"="Cooling event successfully activated", "User Level"=w400, "Value"="True", "Location"="Cooling Event 2", "Level"="Information") -> ("To Screen"=w394:string)  [unwired: 1 in]
                          n261 = local write "Console"(w394) -> ()
                          "Cool 2 Log" <- FALSE
                        }
                      }
                      "Cool Ind 2" <- TRUE
                    }
                  }
                  n262 = case shown="True" w341 {
                    frame False {
                      n263 = local write "Cool Ind 3"(FALSE) -> ()
                    }
                    frame True {
                      n264 = local write "Cooling System"("Cooling cycle 3 - Active") -> ()
                      n265 = local read "Cool 3 Log"() -> (w380:bool)
                      n266 = case shown="True" w380 {
                        frame False {
                        }
                        frame True {
                          n267 = local read "User Level\n(Debug)"() -> (w389:i32)
                          n268 = call "subLogger.vi"("Description"="Cooling event successfully activated", "User Level"=w389, "Value"="True", "Location"="Cooling Event 3", "Level"="Information") -> ("To Screen"=w383:string)  [unwired: 1 in]
                          n269 = local write "Console"(w383) -> ()
                          "Cool 3 Log" <- FALSE
                        }
                      }
                      "Cool Ind 3" <- TRUE
                    }
                  }
                  n270 = case shown="True" w340 {
                    frame False {
                      n271 = local write "Cool Ind 4"(FALSE) -> ()
                    }
                    frame True {
                      n272 = local write "Cooling System"("Cooling cycle 4 - Active") -> ()
                      n273 = local read "Cool 4 Log"() -> (w369:bool)
                      n274 = case shown="True" w369 {
                        frame False {
                        }
                        frame True {
                          n275 = local read "User Level\n(Debug)"() -> (w378:i32)
                          n276 = call "subLogger.vi"("Description"="Cooling event successfully activated", "User Level"=w378, "Value"="True", "Location"="Cooling Event 4", "Level"="Information") -> ("To Screen"=w372:string)  [unwired: 1 in]
                          n277 = local write "Console"(w372) -> ()
                          "Cool 4 Log" <- FALSE
                        }
                      }
                      "Cool Ind 4" <- TRUE
                    }
                  }
                  n278 = local write "Cooling System"("Master cooling online") -> ()
                  "Cooling System Status" <- w338
                }
              }
              n279 = Unflatten From String(type=T2 {"Numeric"=0.0, "Knob"=0.0, "Knob 2"=0.0, "Knob 3"=0.0, TRUE, "bytes to read"=0, "bytes to read 2"=0} ("Cluster"), binary string=w128, error in (no error)=w126) -> (value=w132:T2, error out=w121:errorcluster)  [unwired: 2 in, 1 out]
              n280 = Unbundle(w132) -> ("Numeric"=w111:dbl, "Knob"=w175:dbl, "Knob 2"=w174:dbl, "Knob 3"=w102:dbl, w106:bool, "bytes to read"=w116:u8, "bytes to read 2"=w115:u8)
              "Emergency Cooling" <- w106
              "Watchdog\n(Debug)" <- w116
              "Event Status\n(Debug)" <- w115
              "X-Value\n(Debug)" <- w111
              "Y-Value\n(Debug" <- w175
              "Z-Value\n(Debug)" <- w174
              "Temperature (C)" <- w102
              n281 = Add(x=w116, y=w115) -> (x+y=w118:u8)
              n282 = case shown="3" w118 {
                frame 0, Default {
                  w198 = FALSE
                  w199 = ""
                  w196 = TRUE
                  w200 = FALSE
                  # "Scenario handler based on values send from controller"
                  # "Offline scenario"
                  n283 = local write "Connected"(w200) -> ()
                  n284 = local write "Authorise\nMovement (Debug)"(w200) -> ()
                  n285 = property on="Auth" class="Bool"("Visible"=w200) -> ()  [unwired: 2 in, 2 out]
                  n286 = property on="Auth 2" class="Bool"("Visible"=w200) -> ()  [unwired: 2 in, 2 out]
                  n287 = property on="Login" class="Bool"("Visible"=w196) -> ()  [unwired: 2 in, 2 out]
                  n288 = local write "Connection Log"(w196) -> ()
                  n289 = local write "Local Log"(w196) -> ()
                  n290 = local write "Moved Log"(w196) -> ()
                  n291 = local write "System Status"("System in local mode - Disconnected") -> ()
                  n292 = local write "Username"(w199) -> ()
                  n293 = local write "Password"(w199) -> ()
                  n294 = local read "Disconnect Log"() -> (w197:bool)
                  n295 = case shown="True" w197 {
                    frame False {
                    }
                    frame True {
                      n296 = local read "User Level\n(Debug)"() -> (w203:i32)
                      n297 = call "subLogger.vi"("Description"="Communication not established", "User Level"=w203, "Value"="False", "Location"="System Comms", "Level"="Information") -> ("To Screen"=w202:string)  [unwired: 1 in]
                      n298 = local write "Console"(w202) -> ()
                      "Disconnect Log" <- FALSE
                    }
                  }
                  "Master Warning" <- w198
                  "Self Destruct" <- w198
                  "Local Request" <- w198
                }
                frame 1 {
                  w212 = FALSE
                  w213 = ""
                  w214 = FALSE
                  w210 = TRUE
                  # "Scenario handler based on values send from controller"
                  # "Normal online operation scenario"
                  n299 = local write "Authorise\nMovement (Debug)"(w214) -> ()
                  n300 = property on="Auth" class="Bool"("Visible"=w214) -> ()  [unwired: 2 in, 2 out]
                  n301 = property on="Auth 2" class="Bool"("Visible"=w214) -> ()  [unwired: 2 in, 2 out]
                  n302 = property on="Login" class="Bool"("Visible"=w210) -> ()  [unwired: 2 in, 2 out]
                  n303 = local write "Disconnect Log"(w210) -> ()
                  n304 = local write "Moved Log"(w210) -> ()
                  n305 = local write "System Status"("System in master mode - Connected") -> ()
                  n306 = local write "Username"(w213) -> ()
                  n307 = local write "Password"(w213) -> ()
                  n308 = local write "Local Request"(w212) -> ()
                  n309 = local write "Self Destruct"(w212) -> ()
                  n310 = local write "Master Warning"(w212) -> ()
                  n311 = local read "Connection Log"() -> (w211:bool)
                  n312 = local read "Local Log"() -> (w209:bool)
                  n313 = case shown="True" w211 {
                    frame False {
                    }
                    frame True {
                      n314 = local read "User Level\n(Debug)"() -> (w225:i32)
                      n315 = call "subLogger.vi"("Description"="Communication established", "User Level"=w225, "Value"="True", "Location"="System Comms", "Level"="Information") -> ("To Screen"=w223:string)  [unwired: 1 in]
                      n316 = local write "Console"(w223) -> ()
                      "Connection Log" <- FALSE
                    }
                  }
                  n317 = case shown="False" w209 {
                    frame True {
                    }
                    frame False {
                      n318 = local read "User Level\n(Debug)"() -> (w218:i32)
                      n319 = call "subLogger.vi"("Description"="Local mode request timed out - denied", "User Level"=w218, "Value"="False", "Location"="System Comms", "Level"="Information") -> ("To Screen"=w217:string)  [unwired: 1 in]
                      n320 = local write "Console"(w217) -> ()
                      n321 = local write "Local Log"(TRUE) -> ()
                    }
                  }
                  "Connected" <- w210
                }
                frame 2 {
                  w246 = TRUE
                  w256 = FALSE
                  w247 = TRUE
                  # "Scenario handler based on values send from controller"
                  # "Movement scenario"
                  n322 = local read "User Type\n(Debug)"() -> (w255:string[])
                  n323 = local read "Username"() -> (w254:string)
                  n324 = local read "Password Match\n(Debug)"() -> (w253:string[])
                  n325 = local read "Password"() -> (w252:string)
                  n326 = local write "Cooling\nSwitch"(w256) -> ()
                  n327 = property on="Auth 2" class="Bool"("Visible"=w256) -> ()  [unwired: 2 in, 2 out]
                  n328 = property on="Login" class="Bool"("Visible"=w256) -> ()  [unwired: 2 in, 2 out]
                  n329 = local write "Connected"(w247) -> ()
                  n330 = property on="Auth" class="Bool"("Visible"=w247) -> ()  [unwired: 2 in, 2 out]
                  n331 = call "subLogin.vi"("Login Button"="Auth", "Password Entry"=w252, "Password Array"=w253, "User Entry"=w254, "User Array"=w255) -> ("Array Index No"=w250:i32, "If Correct 2"=w243:bool, "If Correct 1"=w249:bool, "If Incorrect"=w244:bool)  [unwired: 1 out]
                  n332 = Equal?(x=w250, y=3 ("bytes to read")) -> (x = y?=w248:bool)
                  n333 = local write "Master Warning"(w246) -> ()
                  n334 = local write "Self Destruct"(w246) -> ()
                  n335 = case shown="True" w243 {
                    frame True {
                      w265 = "Auth Granted"
                      n336 = local read "User Level\n(Debug)"() -> (w261:i32)
                      n337 = local write "User Status"(w265) -> ()
                      n338 = call "subLogger.vi"("Description"="Authorisation granted", "User Level"=w261, "Value"=w265, "Location"="Auth System", "Level"="Warning") -> ("To Screen"=w260:string)  [unwired: 1 in]
                      n339 = local write "Console"(w260) -> ()
                    }
                    frame False {
                    }
                  }
                  n340 = And(x=w249, y=w248) -> (x .and. y?=w257:bool)
                  n341 = local write "Authorise\nMovement (Debug)"(w257) -> ()
                  n342 = local write "System Status"("Unauthorised movement detected! - Verify Immediately") -> ()
                  n343 = local read "X-Value\n(Debug)"() -> (w237:dbl)
                  n344 = local read "Y-Value\n(Debug"() -> (w240:dbl)
                  n345 = local read "Z-Value\n(Debug)"() -> (w238:dbl)
                  n346 = Format Into String(format string="%.;%.2f", w237) -> (resulting string=w235:string)  [unwired: 2 in, 1 out]
                  n347 = Format Into String(format string="%.;%.2f", w240) -> (resulting string=w233:string)  [unwired: 2 in, 1 out]
                  n348 = Format Into String(format string="%.;%.2f", w238) -> (resulting string=w231:string)  [unwired: 2 in, 1 out]
                  n349 = local read "Moved Log"() -> (w245:bool)
                  n350 = Concatenate Strings("X: ", w235, ", Y: ", w233, ", Z: ", w231) -> (w230:string)
                  n351 = case shown="True" w244 {
                    frame True {
                      w271 = "Auth Failed"
                      n352 = local read "User Level\n(Debug)"() -> (w267:i32)
                      n353 = local write "User Status"(w271) -> ()
                      n354 = call "subLogger.vi"("Description"="Incorrect authorisation attempted", "User Level"=w267, "Value"=w271, "Location"="Login System", "Level"="Warning") -> ("To Screen"=w266:string)  [unwired: 1 in]
                      n355 = local write "Console"(w266) -> ()
                    }
                    frame False {
                    }
                  }
                  n356 = case shown="True" w245 {
                    tunnel: w230 -> [_ w273]
                    frame False {
                    }
                    frame True {
                      n357 = local read "User Level\n(Debug)"() -> (w275:i32)
                      n358 = call "subLogger.vi"("Description"="Movement detected", "User Level"=w275, "Value"=w273, "Location"="Controller Ops", "Level"="Warning") -> ("To Screen"=w272:string)  [unwired: 1 in]
                      n359 = local write "Console"(w272) -> ()
                      "Moved Log" <- FALSE
                    }
                  }
                }
                frame 3 {
                  w282 = TRUE
                  w293 = FALSE
                  w294 = TRUE
                  # "Scenario handler based on values send from controller"
                  # "Local scenario"
                  n360 = local read "User Type\n(Debug)"() -> (w290:string[])
                  n361 = local read "Username"() -> (w289:string)
                  n362 = local read "Password Match\n(Debug)"() -> (w288:string[])
                  n363 = local read "Password"() -> (w287:string)
                  n364 = property on="Login" class="Bool"("Visible"=w293) -> ()  [unwired: 2 in, 2 out]
                  n365 = property on="Auth" class="Bool"("Visible"=w293) -> ()  [unwired: 2 in, 2 out]
                  n366 = local write "Connected"(w294) -> ()
                  n367 = property on="Auth 2" class="Bool"("Visible"=w294) -> ()  [unwired: 2 in, 2 out]
                  n368 = call "subLogin.vi"("Login Button"="Auth 2", "Password Entry"=w287, "Password Array"=w288, "User Entry"=w289, "User Array"=w290) -> ("Array Index No"=w286:i32, "If Correct 2"=w279:bool, "If Correct 1"=w284:bool, "If Incorrect"=w280:bool)  [unwired: 1 out]
                  n369 = local write "Local Request"(w282) -> ()
                  n370 = local write "Master Warning"(w282) -> ()
                  n371 = Equal?(x=w286, y=3 ("bytes to read")) -> (x = y?=w283:bool)
                  n372 = And(x=w284, y=w283) -> (x .and. y?=w292:bool)
                  n373 = local write "Authorise\nMovement (Debug)"(w292) -> ()
                  n374 = case shown="True" w279 {
                    frame True {
                      w301 = "Auth Granted"
                      n375 = local read "User Level\n(Debug)"() -> (w297:i32)
                      n376 = local write "User Status"(w301) -> ()
                      n377 = call "subLogger.vi"("Description"="Authorisation granted", "User Level"=w297, "Value"=w301, "Location"="Auth System", "Level"="Warning") -> ("To Screen"=w296:string)  [unwired: 1 in]
                      n378 = local write "Console"(w296) -> ()
                    }
                    frame False {
                    }
                  }
                  n379 = local write "System Status"("Local mode requested! - Awaiting authorisation") -> ()
                  n380 = local read "Local Log"() -> (w281:bool)
                  n381 = case shown="True" w280 {
                    frame True {
                      w307 = "Auth Failed"
                      n382 = local read "User Level\n(Debug)"() -> (w303:i32)
                      n383 = local write "User Status"(w307) -> ()
                      n384 = call "subLogger.vi"("Description"="Incorrect authorisation attempted", "User Level"=w303, "Value"=w307, "Location"="Auth System", "Level"="Warning") -> ("To Screen"=w302:string)  [unwired: 1 in]
                      n385 = local write "Console"(w302) -> ()
                    }
                    frame False {
                    }
                  }
                  n386 = case shown="True" w281 {
                    frame False {
                    }
                    frame True {
                      n387 = local read "User Level\n(Debug)"() -> (w310:i32)
                      n388 = call "subLogger.vi"("Description"="Local mode request received", "User Level"=w310, "Value"="True", "Location"="Controller Ops", "Level"="Information") -> ("To Screen"=w308:string)  [unwired: 1 in]
                      n389 = local write "Console"(w308) -> ()
                      "Local Log" <- FALSE
                    }
                  }
                }
                frame 4 {
                  w316 = TRUE
                  w317 = FALSE
                  # "Scenario handler based on values send from controller"
                  # "Self destruct scenario"
                  n390 = property on="Login" class="Bool"("Visible"=w317) -> ()  [unwired: 2 in, 2 out]
                  n391 = property on="Auth" class="Bool"("Visible"=w317) -> ()  [unwired: 2 in, 2 out]
                  n392 = property on="Auth 2" class="Bool"("Visible"=w317) -> ()  [unwired: 2 in, 2 out]
                  n393 = local write "Connected"(w317) -> ()
                  n394 = local write "Local Request"(w317) -> ()
                  n395 = local write "Master Warning"(w316) -> ()
                  n396 = local write "Self Destruct"(w316) -> ()
                  n397 = local write "System Status"("Self Destruct - Controller Destroyed!") -> ()
                  n398 = local read "Destroyed Log"() -> (w315:bool)
                  n399 = case shown="True" w315 {
                    frame False {
                    }
                    frame True {
                      n400 = local read "User Level\n(Debug)"() -> (w321:i32)
                      n401 = call "subLogger.vi"("Description"="Controller reported destroyed!", "User Level"=w321, "Value"="True", "Location"="System Comms", "Level"="Warning") -> ("To Screen"=w319:string)  [unwired: 1 in]
                      n402 = local write "Console"(w319) -> ()
                      "Destroyed Log" <- FALSE
                    }
                  }
                }
              }
              n403 = Bundle("Numeric"=w111, "Knob"=w175, "Knob 2"=w174) -> (→"Movement":cluster{"Numeric":dbl, "Knob":dbl, "Knob 2":dbl})  [unwired: 1 in]
              n404 = Not(x=w106) -> (.not. x?=w107:bool)
              "Safe System Temperature" <- w107
              n405 = local read "Cooling Event Array\n(Debug)"() -> (w158:bool[])
              n406 = local read "Cool Ind 1"() -> (w163:bool)
              n407 = local read "Cool Ind 2"() -> (w162:bool)
              n408 = local read "Cool Ind 3"() -> (w161:bool)
              n409 = local read "Cool Ind 4"() -> (w160:bool)
              n410 = Build Array(w163, w162, w161, w160) -> (→"Cooling Event Array\n(Debug)":bool[])
              n411 = Or Array Elements(Boolean array=w158) -> (logical OR=w164:bool)
              n412 = Select(t=0.1, s=w164, f=0.05) -> (s? t:f=w167:dbl)
              n413 = Bundle("Cool Ind 1"=w163, "Cool Ind 2"=w162, "Cool Ind 3"=w161, "Cool Ind 4"=w160, w164, w167, "Authorise\nMovement (Debug)"="Authorise\nMovement (Debug)") -> (w125:T4)  [unwired: 1 in]
              n414 = Flatten To String(anything=w125, error in (no error)=w121) -> (data string=w124:string, error out=w120:errorcluster)  [unwired: 2 in, 1 out]
              n415 = String Length(string=w124) -> (length=w123:i32)
              "String Length\n(Debug)" <- w123
              n416 = Flatten To String(anything=w123, error in (no error)=w120) -> (data string=w122:string, error out=w119:errorcluster)  [unwired: 2 in, 1 out]
              n417 = TCP Write(connection ID=w171, data in=w122, error in (no error)=w119) -> (connection ID out=w170:refnum<k5>, bytes written=→"Data Size\n(Debug)":i32, error out=w172:errorcluster)  [unwired: 1 out]
              n418 = TCP Write(connection ID=w170, data in=w124, error in (no error)=w172) -> (connection ID out=w151:refnum<k5>, error out=w140:errorcluster)  [unwired: 2 out]
              n419 = local read "Nom Temp Log"() -> (w108:bool)
              n420 = local read "High Temp Log"() -> (w105:bool)
              n421 = Format Into String(format string="%.;%.2f", w102) -> (resulting string=w112:string)  [unwired: 2 in, 1 out]
              n422 = And(x=w107, y=w108) -> (x .and. y?=w109:bool)
              n423 = And(x=w106, y=w105) -> (x .and. y?=w110:bool)
              n424 = case shown="True" w109 {
                tunnel: w112 -> [_ w190]
                frame False {
                }
                frame True {
                  n425 = local read "User Level\n(Debug)"() -> (w192:i32)
                  n426 = call "subLogger.vi"("Clear Flag"=FALSE, "Description"="Temperature range nominal", "User Level"=w192, "Value"=w190, "Location"="Controller Ops", "Level"="Information") -> ("To Screen"=w188:string)
                  n427 = local write "Console"(w188) -> ()
                  n428 = local write "High Temp Log"(TRUE) -> ()
                  "Nom Temp Log" <- FALSE
                }
              }
              n429 = case shown="True" w110 {
                tunnel: w112 -> [_ w181]
                frame False {
                }
                frame True {
                  n430 = local read "User Level\n(Debug)"() -> (w183:i32)
                  n431 = call "subLogger.vi"("Clear Flag"=FALSE, "Description"="Temperature range high!", "User Level"=w183, "Value"=w181, "Location"="Controller Ops", "Level"="Warning") -> ("To Screen"=w179:string)
                  n432 = local write "Console"(w179) -> ()
                  n433 = local write "Nom Temp Log"(TRUE) -> ()
                  "High Temp Log" <- FALSE
                }
              }
              n434 = Unbundle By Name(w140) -> ("status"=w139:bool)
              n435 = local read "Quit"() -> (w146:bool)
              n436 = Unbundle(w140) -> ("status"=→"Net Error Status\n(Debug)":bool, "code"=→"Net Error Code\n(Debug)":i32, "source"=→"Net Error Source\n(Debug)":string)
              n437 = Or(x=w146, y="Log Off") -> (x .or. y?=w141:bool)
              n438 = call <vilib>:"Simple Error Handler.vi"("type of dialog (OK msg:1)"=u16 0, "error in (no error)"=w140) -> ("code out"=→"Handler Error Code\n(Debug)":i32, "error out"=w152:errorcluster)  [unwired: 6 out]
              n439 = Or(x=w139, y=w141) -> (x .or. y?=w138:bool)
              n440 = Wait (ms)(milliseconds to wait=u32 100) -> ()  [unwired: 1 out]
            }
            n441 = TCP Close Connection(connection ID=w94, error in (no error)=w95) -> (error out=w74:errorcluster)  [unwired: 2 out]
            n442 = call "IMAQ Dispose"("Image"=w90) -> ("error out"=w86:errorcluster)  [unwired: 5 in]
            n443 = Unbundle By Name(w74) -> ("code"=w73:i32)
            n444 = local read "User Level\n(Debug)"() -> (w75:i32)
            n445 = call <vilib>:"Simple Error Handler.vi"("error in (no error)"=w86) -> ()  [unwired: 1 in, 8 out]
            n446 = Number To Decimal String(number=w73) -> (decimal integer string=w79:string)  [unwired: 1 in]
            n447 = call "subLogger.vi"("Description"="Network disconnection", "User Level"=w75, "Value"=w79, "Location"="TCP", "Level"="Information") -> ("To Screen"=w71:string)  [unwired: 1 in]
            n448 = local write "Console"(w71) -> ()
            n449 = call <vilib>:"Error to Warning.vi"("1st Error to Convert"=w98, "2nd Error to Convert"=w97, "3rd Error to Convert"=w96, "4th Error to Convert"=w92, "error in"=w74) -> ()  [unwired: 1 in, 10 out]
            "User Level\n(Debug)" <- w81
          }
        }
        "User Status" <- "Logged Out"
        "Cooling System" <- "Master cooling offline"
      }
    }
    frame #2 {
      w418 = FALSE
      w419 = TRUE
      w421 = FALSE
      w422 = FALSE
      w420 = FALSE
      w428 = TRUE
      w417 = 0.0 ("Numeric")
      w429 = ""
      # "Show login button"
      # "Log close down"
      # "Clear lights"
      # "Enable Log Systems"
      # "Hide log indicators"
      # "Hide debug controls"
      # "Hide user controls"
      # "Enable cooling"
      # "Set system status"
      # "Clear indicators"
      # "Clear log in fields"
      n450 = local write "Cool System On Log"(w419) -> ()
      n451 = local write "Cool 4 Log"(w419) -> ()
      n452 = local write "Cool 3 Log"(w419) -> ()
      n453 = local write "Cool 2 Log"(w419) -> ()
      n454 = local write "Cool 1 Log"(w419) -> ()
      n455 = local write "Destroyed Log"(w419) -> ()
      n456 = local write "Local Log"(w419) -> ()
      n457 = local write "Moved Log"(w419) -> ()
      n458 = local write "Disconnect Log"(w419) -> ()
      n459 = local write "Connection Log"(w419) -> ()
      n460 = local write "Nom Temp Log"(w419) -> ()
      n461 = local write "High Temp Log"(w419) -> ()
      n462 = local write "Cool System Off Log"(w419) -> ()
      n463 = local write "Cool System On Log"(w419) -> ()
      n464 = local write "Local Log"(w419) -> ()
      n465 = local write "Moved Log"(w419) -> ()
      n466 = local write "Emergency Cooling"(w418) -> ()
      n467 = local write "Safe System Temperature"(w418) -> ()
      n468 = local write "Connected"(w418) -> ()
      n469 = local write "Local Request"(w418) -> ()
      n470 = local write "Self Destruct"(w418) -> ()
      n471 = local write "Master Warning"(w418) -> ()
      n472 = local write "Quit"(w418) -> ()
      n473 = property on="Cooling 1 On" class="AbsTime (strict)"("Visible"=w420) -> ()  [unwired: 2 in, 2 out]
      n474 = property on="Cooling 1 Off" class="AbsTime (strict)"("Visible"=w420) -> ()  [unwired: 2 in, 2 out]
      n475 = property on="Cooling 2 On" class="AbsTime (strict)"("Visible"=w420) -> ()  [unwired: 2 in, 2 out]
      n476 = property on="Cooling 2 Off" class="AbsTime (strict)"("Visible"=w420) -> ()  [unwired: 2 in, 2 out]
      n477 = property on="Cooling 3 On" class="AbsTime (strict)"("Visible"=w420) -> ()  [unwired: 2 in, 2 out]
      n478 = property on="Cooling 3 Off" class="AbsTime (strict)"("Visible"=w420) -> ()  [unwired: 2 in, 2 out]
      n479 = property on="Cooling 4 On" class="AbsTime (strict)"("Visible"=w420) -> ()  [unwired: 2 in, 2 out]
      n480 = property on="Cooling 4 Off" class="AbsTime (strict)"("Visible"=w420) -> ()  [unwired: 2 in, 2 out]
      n481 = property on="Cooling\nSwitch" class="Bool (strict)"("Visible"=w420) -> ()  [unwired: 2 in, 2 out]
      n482 = local write "Cooling\nSwitch"(w428) -> ()
      n483 = property on="Login" class="Bool"("Visible"=w428) -> ()  [unwired: 2 in, 2 out]
      n484 = call "subLogger.vi"("Description"="Closing system", "User Level"=-1, "Value"="True", "Location"="Service Shutdown", "Level"="Information") -> ()  [unwired: 1 in, 1 out]
      n485 = property on="Cooling Light 1" class="Bool (strict)"("Visible"=w420) -> ()  [unwired: 2 in, 2 out]
      n486 = property on="Cooling Light 2" class="Bool (strict)"("Visible"=w420) -> ()  [unwired: 2 in, 2 out]
      n487 = property on="Cooling Light 3" class="Bool (strict)"("Visible"=w420) -> ()  [unwired: 2 in, 2 out]
      n488 = property on="Cooling Light 4" class="Bool (strict)"("Visible"=w420) -> ()  [unwired: 2 in, 2 out]
      n489 = property on="Cooling System Status" class="Bool (strict)"("Visible"=w420) -> ()  [unwired: 2 in, 2 out]
      n490 = property on="Auth 2" class="Bool"("Visible"=w420) -> ()  [unwired: 2 in, 2 out]
      n491 = property on="Auth" class="Bool"("Visible"=w420) -> ()  [unwired: 2 in, 2 out]
      n492 = local write "Password"(w429) -> ()
      n493 = local write "Username"(w429) -> ()
      n494 = Bundle("Numeric"=w417, "Numeric"=w417, "Numeric"=w417) -> (w431:T3)  [unwired: 1 in]
      n495 = local write "Temperature (C)"(w417) -> ()
      n496 = local write "System Status"("System Offline") -> ()
      n497 = local write "Movement"(w431) -> ()
      n498 = property on="Cooling Event Array\n(Debug)" class="Arr (strict)"("Visible"=w421) -> ()  [unwired: 2 in, 2 out]
      n499 = property on="String Length\n(Debug)" class="DigNum (strict)"("Visible"=w421) -> ()  [unwired: 2 in, 2 out]
      n500 = property on="Data Size\n(Debug)" class="DigNum (strict)"("Visible"=w421) -> ()  [unwired: 2 in, 2 out]
      n501 = property on="Net Error Status\n(Debug)" class="Bool (strict)"("Visible"=w421) -> ()  [unwired: 2 in, 2 out]
      n502 = property on="Handler Error Code\n(Debug)" class="DigNum (strict)"("Visible"=w421) -> ()  [unwired: 2 in, 2 out]
      n503 = property on="User Level\n(Debug)" class="DigNum (strict)"("Visible"=w421) -> ()  [unwired: 2 in, 2 out]
      n504 = property on="Cool 1 Log" class="Bool (strict)"("Visible"=w422) -> ()  [unwired: 2 in, 2 out]
      n505 = property on="Cool 2 Log" class="Bool (strict)"("Visible"=w422) -> ()  [unwired: 2 in, 2 out]
      n506 = property on="Cool 3 Log" class="Bool (strict)"("Visible"=w422) -> ()  [unwired: 2 in, 2 out]
      n507 = property on="Cool 4 Log" class="Bool (strict)"("Visible"=w422) -> ()  [unwired: 2 in, 2 out]
      n508 = property on="Cool System On Log" class="Bool (strict)"("Visible"=w422) -> ()  [unwired: 2 in, 2 out]
      n509 = property on="Cool System Off Log" class="Bool (strict)"("Visible"=w422) -> ()  [unwired: 2 in, 2 out]
      n510 = property on="Nom Temp Log" class="Bool (strict)"("Visible"=w422) -> ()  [unwired: 2 in, 2 out]
      n511 = property on="High Temp Log" class="Bool (strict)"("Visible"=w422) -> ()  [unwired: 2 in, 2 out]
      n512 = property on="Connection Log" class="Bool (strict)"("Visible"=w422) -> ()  [unwired: 2 in, 2 out]
      n513 = property on="Net Error Source\n(Debug)" class="Str"("Visible"=w421) -> ()  [unwired: 2 in, 2 out]
      n514 = property on="Authorise\nMovement (Debug)" class="Bool (strict)"("Visible"=w421) -> ()  [unwired: 2 in, 2 out]
      n515 = property on="Watchdog\n(Debug)" class="DigNum (strict)"("Visible"=w421) -> ()  [unwired: 2 in, 2 out]
      n516 = property on="Net Error Code\n(Debug)" class="DigNum (strict)"("Visible"=w421) -> ()  [unwired: 2 in, 2 out]
      n517 = property on="User Type\n(Debug)" class="Arr (strict)"("Visible"=w421) -> ()  [unwired: 2 in, 2 out]
      n518 = property on="Password Match\n(Debug)" class="Arr (strict)"("Visible"=w421) -> ()  [unwired: 2 in, 2 out]
      n519 = property on="Moved Log" class="Bool (strict)"("Visible"=w422) -> ()  [unwired: 2 in, 2 out]
      n520 = property on="Disconnect Log" class="Bool (strict)"("Visible"=w422) -> ()  [unwired: 2 in, 2 out]
      n521 = property on="Destroyed Log" class="Bool (strict)"("Visible"=w422) -> ()  [unwired: 2 in, 2 out]
      n522 = property on="Local Log" class="Bool (strict)"("Visible"=w422) -> ()  [unwired: 2 in, 2 out]
      n523 = property on="Cool System Off Log" class="Bool (strict)"("Visible"=w422) -> ()  [unwired: 2 in, 2 out]
      n524 = property on="Event Status\n(Debug)" class="DigNum (strict)"("Visible"=w421) -> ()  [unwired: 2 in, 2 out]
      n525 = property on="X-Value\n(Debug)" class="DigNum (strict)"("Visible"=w421) -> ()  [unwired: 2 in, 2 out]
      n526 = property on="Y-Value\n(Debug" class="DigNum (strict)"("Visible"=w421) -> ()  [unwired: 2 in, 2 out]
      n527 = property on="Z-Value\n(Debug)" class="DigNum (strict)"("Visible"=w421) -> ()  [unwired: 2 in, 2 out]
    }
  }
